vi "DSF.Memory.Cache.Transfer.Get Buffer.vi"(8 "error in (no error)":errorcluster, 11 "Transfer Cache in":refnum<class "DSF.Memory.Cache.Transfer.lvclass">) -> (0 "error out":errorcluster, 2 "Buffer":refnum<class "DSF.Memory.Buffer.lvclass">, 3 "Transfer Cache out":refnum<class "DSF.Memory.Cache.Transfer.lvclass">)   [LabVIEW 2016, in "DSF.Memory.lvlib" / "DSF.Memory.Cache.Transfer.lvclass"]
uses:
  DSF.Memory.Cache.Transfer.lvclass
  Memory.Buffer/DSF.Memory.Buffer.lvclass
  DSF.Memory.Cache.Transfer.lvclass/DSF.Memory.Cache.Transfer.ctl
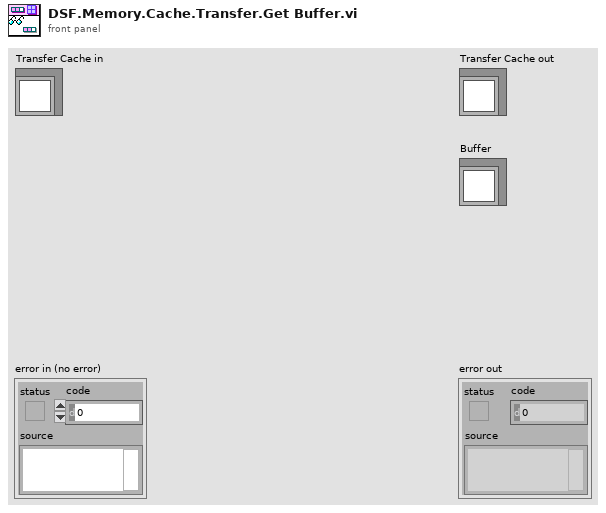
[diagram p1: front panel]
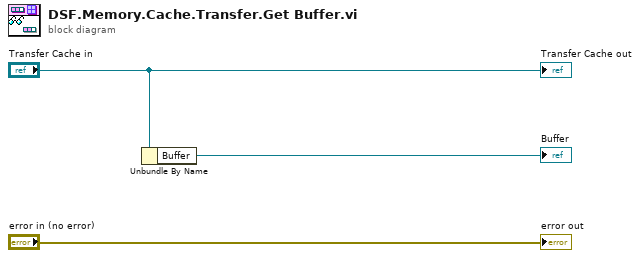
[diagram p0: block diagram]
diagram:
  n1 = Unbundle By Name("Transfer Cache in") -> ("Buffer"=→"Buffer":refnum<class "DSF.Memory.Buffer.lvclass">)
  "error out" <- "error in (no error)"
  "Transfer Cache out" <- "Transfer Cache in"
